vi "Exercise 10.2_Answer.vi"() -> ()   [LabVIEW 2010]
panel:
  in  "Stop":bool
  out "Walk Sign":bool
  out "Green":bool
  out "Yellow":bool
  out "Red":bool
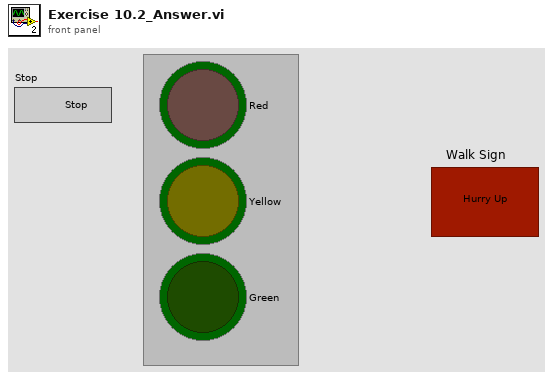
[diagram p1: front panel]
types:
  T1 = enum16{"Initialize", "Green", "Yellow", "Red 1", "Red 2", "Stop"}
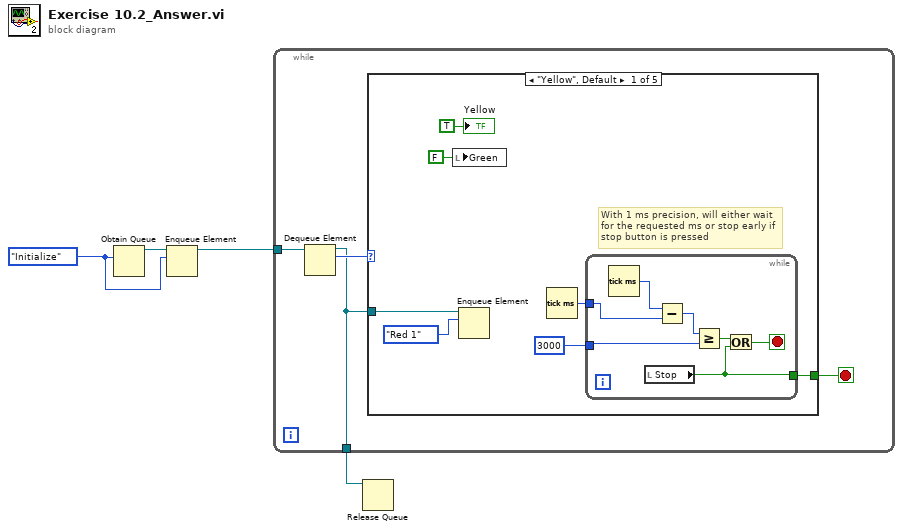
[diagram p0: block diagram]
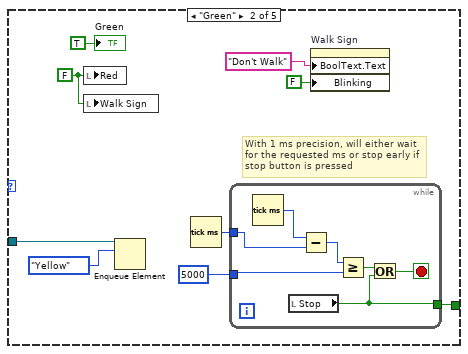
[diagram p2: hidden frame]
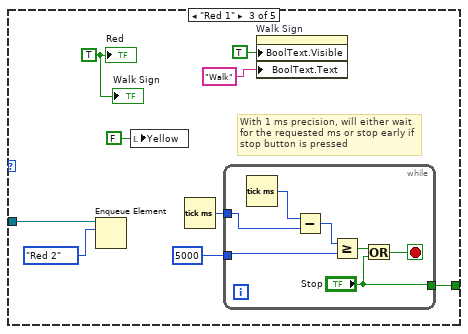
[diagram p3: hidden frame]
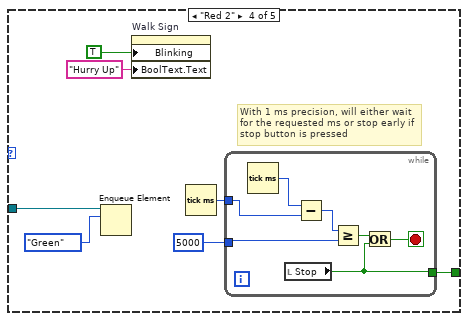
[diagram p4: hidden frame]
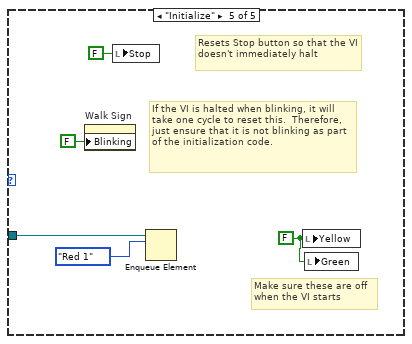
[diagram p5: hidden frame]
diagram:
  w2 = T1."Initialize"
  n1 = Obtain Queue(element data type=w2) -> (queue out=w4:refnum<queue>)  [unwired: 4 in, 2 out]
  n2 = Enqueue Element(queue=w4, element=w2) -> (queue out=w3:refnum<queue>)  [unwired: 2 in, 2 out]
  n3 = while {
    tunnel: w3 -> [w8]
    tunnel: [w5] -> w1
    stop <- w6 stop-if-true
    n4 = Dequeue Element(queue=w8) -> (queue out=w5:refnum<queue>, element=w7:T1)  [unwired: 2 in, 2 out]
    n5 = case shown="\"Yellow\", Default" w7 {
      tunnel: w5 -> [w9 w26 w41 w58 w71]
      tunnel: [w13 w23 w39 w55 _] -> w6
      frame "Yellow", Default {
        # "With 1 ms precision, will either wait for the requested ms or stop early if stop button is pressed"
        n6 = local write "Green"(FALSE ("Green")) -> ()
        n7 = Enqueue Element(queue=w9, element=T1."Red 1") -> ()  [unwired: 2 in, 3 out]
        n8 = Tick Count (ms)() -> (millisecond timer value=w15:u32)
        n9 = while {
          tunnel: w15 -> [w21]
          tunnel: u32 3000 ("milliseconds to wait") -> [w19]
          tunnel: [w16] -> w13
          stop <- w17 stop-if-true
          n10 = Tick Count (ms)() -> (millisecond timer value=w22:u32)
          n11 = local read "Stop"() -> (w16:bool)
          n12 = Subtract(x=w22, y=w21) -> (x-y=w20:u32)
          n13 = Greater Or Equal?(x=w20, y=w19) -> (x >= y?=w18:bool)
          n14 = Or(x=w18, y=w16) -> (x .or. y?=w17:bool)
        }
        "Yellow" <- TRUE ("Yellow")
      }
      frame "Green" {
        w31 = FALSE ("Red")
        # "With 1 ms precision, will either wait for the requested ms or stop early if stop button is pressed"
        n15 = local write "Red"(w31) -> ()
        n16 = local write "Walk Sign"(w31) -> ()
        n17 = Enqueue Element(queue=w26, element=T1."Yellow") -> ()  [unwired: 2 in, 3 out]
        n18 = Tick Count (ms)() -> (millisecond timer value=w25:u32)
        n19 = while {
          tunnel: w25 -> [w37]
          tunnel: u32 5000 ("milliseconds to wait") -> [w35]
          tunnel: [w32] -> w23
          stop <- w33 stop-if-true
          n20 = Tick Count (ms)() -> (millisecond timer value=w38:u32)
          n21 = local read "Stop"() -> (w32:bool)
          n22 = Subtract(x=w38, y=w37) -> (x-y=w36:u32)
          n23 = Greater Or Equal?(x=w36, y=w35) -> (x >= y?=w34:bool)
          n24 = Or(x=w34, y=w32) -> (x .or. y?=w33:bool)
        }
        n25 = property on="Walk Sign" class="Bool"("BoolText.Text"="Don't Walk" ("Boolean Text.Text"), "Blinking"=FALSE) -> ()  [unwired: 2 in, 2 out]
        "Green" <- TRUE ("Green")
      }
      frame "Red 1" {
        w47 = TRUE ("Red")
        # "With 1 ms precision, will either wait for the requested ms or stop early if stop button is pressed"
        n26 = Enqueue Element(queue=w41, element=T1."Red 2") -> ()  [unwired: 2 in, 3 out]
        n27 = local write "Yellow"(FALSE ("Yellow")) -> ()
        n28 = Tick Count (ms)() -> (millisecond timer value=w43:u32)
        n29 = while {
          tunnel: w43 -> [w53]
          tunnel: u32 5000 ("milliseconds to wait") -> [w51]
          tunnel: ["Stop"] -> w39
          stop <- w49 stop-if-true
          n30 = Tick Count (ms)() -> (millisecond timer value=w54:u32)
          n31 = Subtract(x=w54, y=w53) -> (x-y=w52:u32)
          n32 = Greater Or Equal?(x=w52, y=w51) -> (x >= y?=w50:bool)
          n33 = Or(x=w50, y="Stop") -> (x .or. y?=w49:bool)
        }
        n34 = property on="Walk Sign" class="Bool"("BoolText.Visible"=TRUE ("Boolean Text.Visible"), "BoolText.Text"="Walk" ("Boolean Text.Text")) -> ()  [unwired: 2 in, 2 out]
        "Red" <- w47
        "Walk Sign" <- w47
      }
      frame "Red 2" {
        # "With 1 ms precision, will either wait for the requested ms or stop early if stop button is pressed"
        n35 = Enqueue Element(queue=w58, element=T1."Green") -> ()  [unwired: 2 in, 3 out]
        n36 = property on="Walk Sign" class="Bool"("Blinking"=TRUE, "BoolText.Text"="Hurry Up" ("Boolean Text.Text")) -> ()  [unwired: 2 in, 2 out]
        n37 = Tick Count (ms)() -> (millisecond timer value=w57:u32)
        n38 = while {
          tunnel: w57 -> [w67]
          tunnel: u32 5000 ("milliseconds to wait") -> [w65]
          tunnel: [w62] -> w55
          stop <- w63 stop-if-true
          n39 = Tick Count (ms)() -> (millisecond timer value=w68:u32)
          n40 = local read "Stop"() -> (w62:bool)
          n41 = Subtract(x=w68, y=w67) -> (x-y=w66:u32)
          n42 = Greater Or Equal?(x=w66, y=w65) -> (x >= y?=w64:bool)
          n43 = Or(x=w64, y=w62) -> (x .or. y?=w63:bool)
        }
      }
      frame "Initialize" {
        w69 = FALSE ("Yellow")
        # "Make sure these are off\nwhen the VI starts"
        # "Resets Stop button so that the VI doesn't immediately halt"
        # "If the VI is halted when blinking, it will take one cycle to reset this.  Therefore, just ensure that it is not blinking as part of the initialization code."
        n44 = property on="Walk Sign" class="Bool"("Blinking"=FALSE) -> ()  [unwired: 2 in, 2 out]
        n45 = local write "Stop"(FALSE ("Stop")) -> ()
        n46 = Enqueue Element(queue=w71, element=T1."Red 1") -> ()  [unwired: 2 in, 3 out]
        n47 = local write "Yellow"(w69) -> ()
        n48 = local write "Green"(w69) -> ()
      }
    }
  }
  n49 = Release Queue(queue=w1) -> ()  [unwired: 2 in, 3 out]
